vi "Create Date-Time file.vi"(0 "File name":string, 5 "Desired path":string, 11 "error in (no error)":errorcluster) -> (4 "Path and name":path, 15 "error out":errorcluster)   [LabVIEW 2018]
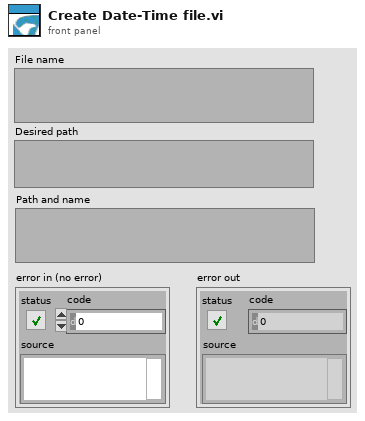
[diagram p1: front panel]
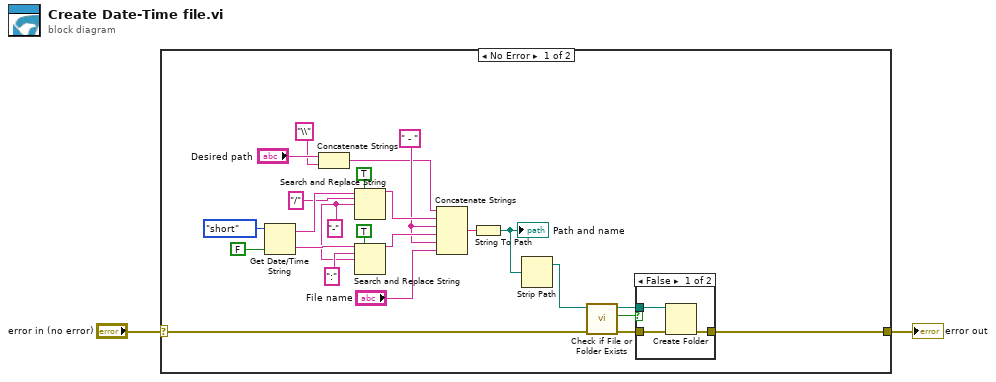
[diagram p0: block diagram]
diagram:
  n1 = case shown="No Error" "error in (no error)" {
    selector: "error in (no error)" -> [w6 w31]
    tunnel: [w7 w31] -> w1
    frame No Error {
      w13 = "-" ("string")
      w18 = " - " ("string")
      n2 = Get Date/Time String(date format (0)=enum16{"short", "long", "abbreviated"}."short", want seconds? (F)=FALSE) -> (date string=w12:string, time string=w15:string)  [unwired: 1 out]
      n3 = Concatenate Strings("Desired path", "\\" ("search string")) -> (w3:string)
      n4 = Search and Replace String(replace all?=TRUE ("replace all? (F)"), input string=w12, search string="/", replace string=w13) -> (result string=w19:string)  [unwired: 1 in, 6 out]
      n5 = Search and Replace String(replace all?=TRUE ("replace all? (F)"), input string=w15, search string=":", replace string=w13) -> (result string=w20:string)  [unwired: 1 in, 6 out]
      n6 = Concatenate Strings(w3, w19, w18, w20, w18, "File name") -> (w10:string)
      n7 = String To Path(string=w10) -> (path=w22:path)
      "Path and name" <- w22
      n8 = Strip Path(path=w22) -> (stripped path=w23:path)  [unwired: 1 out]
      n9 = call <vilib>:"Check if File or Folder Exists.vi"("error in (no error)"=w6, "path"=w23) -> ("error out"=w26:errorcluster, "file or folder exists?"=w25:bool, "dup path"=w24:path)  [unwired: 7 in]
      n10 = case shown="False" w25 {
        tunnel: w24 -> [w29 _]
        tunnel: [w28 w30] -> w7
        tunnel: w26 -> [w27 w30]
        frame False {
          n11 = Create Folder(path (use dialog)=w29, error in=w27) -> (error out=w28:errorcluster)  [unwired: 1 in, 2 out]
        }
        frame True {
        }
      }
    }
    frame Error {
    }
  }
  "error out" <- w1
